vi "init_imaq_images.vi"(8 "error in (no error)":errorcluster) -> (0 "error out":errorcluster, 2 "Resolution":cluster{"X Resolution":i32, "Y Resolution":i32}, 3 "Images":T1[](array[typedef]))   [LabVIEW 2013, in "subVIs.lvlib"]
uses:
  <vilib>/vision/Image Controls.llb/IMAQ Image.ctl
  NI PROJECT/lw project/subVIs.lvlib
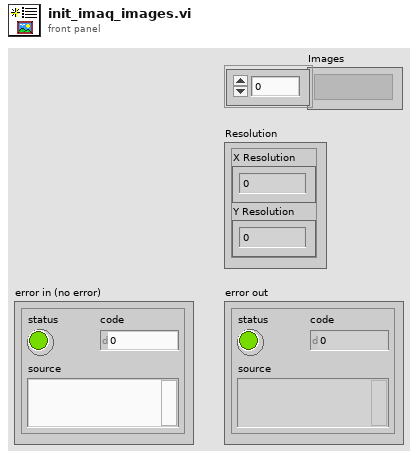
[diagram p1: front panel]
types:
  T1 = typedef "IMAQ Image.ctl" = refnum<image>
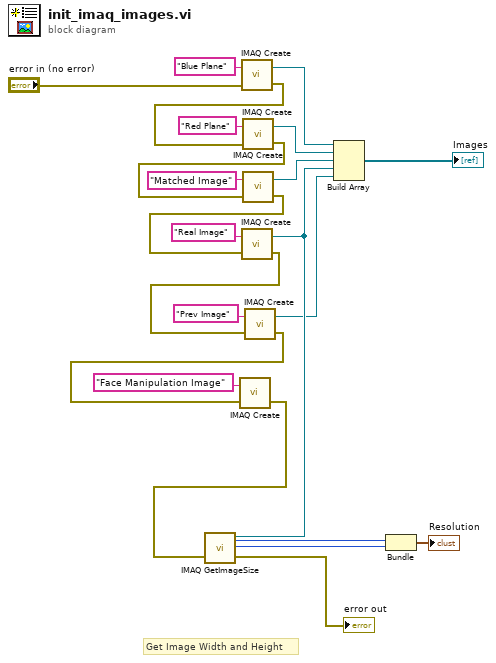
[diagram p0: block diagram]
diagram:
  # "Get Image Width and Height"
  n1 = call "IMAQ Create"("Image Name"="Blue Plane", "error in (no error)"="error in (no error)") -> ("New Image"=w15:T1, "error out"=w12:errorcluster)  [unwired: 2 in, 1 out]
  n2 = call "IMAQ Create"("Image Name"="Red Plane", "error in (no error)"=w12) -> ("New Image"=w16:T1, "error out"=w13:errorcluster)  [unwired: 2 in, 1 out]
  n3 = call "IMAQ Create"("Image Name"="Matched Image", "error in (no error)"=w13) -> ("New Image"=w17:T1, "error out"=w14:errorcluster)  [unwired: 2 in, 1 out]
  n4 = call "IMAQ Create"("Image Name"="Real Image", "error in (no error)"=w14) -> ("New Image"=w19:T1, "error out"=w5:errorcluster)  [unwired: 2 in, 1 out]
  n5 = call "IMAQ Create"("Image Name"="Prev Image", "error in (no error)"=w5) -> ("New Image"=w4:T1, "error out"=w1:errorcluster)  [unwired: 2 in, 1 out]
  n6 = call "IMAQ Create"("Image Name"="Face Manipulation Image", "error in (no error)"=w1) -> ("error out"=w2:errorcluster)  [unwired: 2 in, 2 out]
  n7 = call "IMAQ GetImageSize"("Image"=w19, "error in (no error)"=w2) -> ("Y Resolution"=w22:i32, "X Resolution"=w21:i32, "error out"=→"error out":errorcluster)  [unwired: 2 in]
  n8 = Build Array(w15, w16, w17, w19, w4) -> (→"Images":T1[])
  n9 = Bundle("X Resolution"=w21, "Y Resolution"=w22) -> (→"Resolution":cluster{"X Resolution":i32, "Y Resolution":i32})  [unwired: 1 in]
